vi "ConfigChecker.vi"() -> ()   [LabVIEW 2014]
panel:
  out "Should Stop?":bool
  out "Extra Lines Removed":string[](array[string])
  out "result string":string
  out "NonSensed":string[](array[string])
  in  "Auto Config File":path=path "C:/Users/Matthew/Desktop/Auto Config Testing/autoexample.txt"
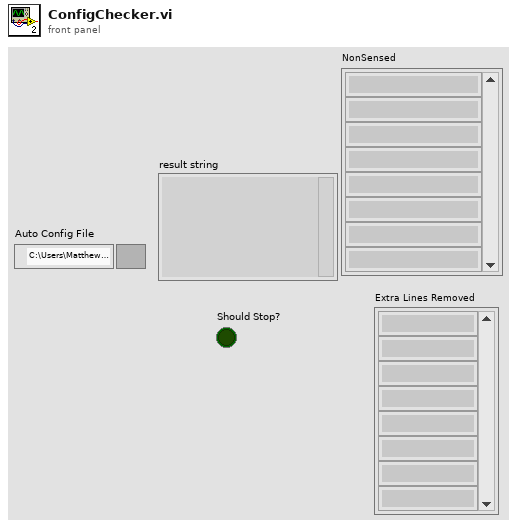
[diagram p1: front panel]
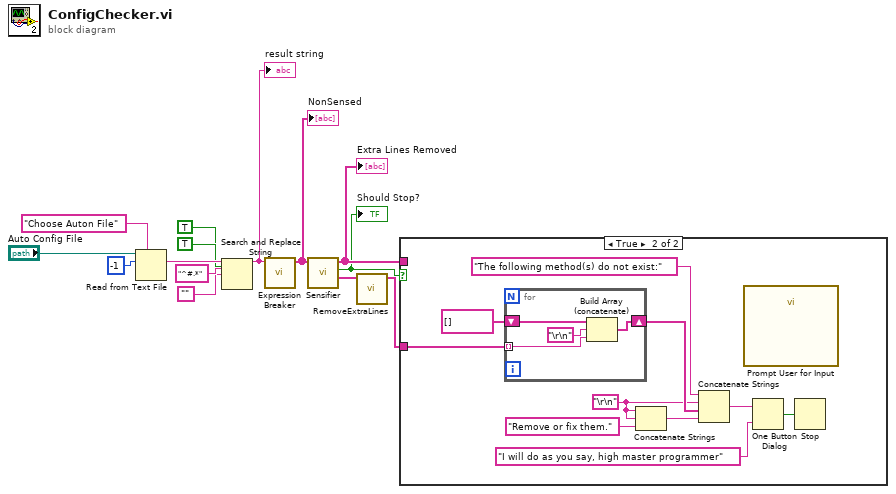
[diagram p0: block diagram]
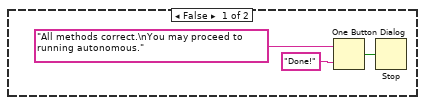
[diagram p2: hidden frame]
diagram:
  n1 = Read from Text File(prompt (Open existing file)="Choose Auton File", file (use dialog)="Auto Config File", count=-1) -> (text=w12:string)  [unwired: 1 in, 3 out]
  n2 = Search and Replace String(replace all?=TRUE ("replace all? (F)"), multiline?=TRUE ("multiline? (F)"), input string=w12, search string="^#.*" ("regular expression"), replace string="") -> (result string=w7:string)  [unwired: 3 in, 3 out]
  "result string" <- w7
  n3 = call "Expression Breaker.vi"("result string"=w7) -> ("Array"=w6:string[])  [unwired: 10 in]
  "NonSensed" <- w6
  n4 = call "Sensifier.vi"("Array"=w6) -> ("Removed Strings"=w5:string[], "Has Errors?"=w2:bool, "Sensed"=w3:string[])  [unwired: 8 in]
  "Extra Lines Removed" <- w3
  "Should Stop?" <- w2
  n5 = call "RemoveExtraLines.vi"("Sensed"=w5) -> ("Output"=w4:string[])  [unwired: 10 in]
  n6 = case shown="True" w2 {
    tunnel: w4 -> [_ w22]
    tunnel: w3 -> [_ _]
    frame False {
      n7 = One Button Dialog(message="All methods correct.\nYou may proceed to running autonomous.", button name ("OK")="Done!") -> (true=w17:bool)
      n8 = Stop(stop? (T)=w17) -> ()
    }
    frame True {
      w19 = "\r\n"
      n9 = for {
        shift-right: [w31] -> w27
        shift-left: string[] [] -> [w28]
        tunnel: w22 -> [w30] mode=indexing
        n10 = Build Array (concatenate)(w28, "\r\n", w30) -> (w31:string[])
      }
      n11 = Concatenate Strings(w19, w19, "Remove or fix them.") -> (w23:string)
      n12 = Concatenate Strings("The following method(s) do not exist:", w19, w27, w23) -> (w26:string)
      n13 = call "Prompt User for Input"() -> ()  [unwired: 18 in, 2 out]
      n14 = One Button Dialog(message=w26, button name ("OK")="I will do as you say, high master programmer") -> (true=w25:bool)
      n15 = Stop(stop? (T)=w25) -> ()
    }
  }
